vi "SLSC Get EDS Module Information_O2.vi"(5 "Password":string, 7 "Username":string="admin", 8 "error in (no error)":errorcluster, 10 "Slot #":u32=6, 11 "Chassis IP Address":string="192.168.8.130") -> (0 "error out":errorcluster, 1 "SLSC Module Name":string, 2 "Initialized?":bool, 3 "SLSC EDS module":T1)   [LabVIEW 2017]
doc: "This vi reads device tree from online SLSC module. If there is no connection possible it reads from a capabilities NVMEM .bin file. Then it creates a cluster containing the whole module tree."
uses:
  SLSC EDS API/JSON parsing/EDSjsonStructure.ctl
  SLSC EDS API/JSON parsing/enum.ctl
  SLSC EDS API/JSON parsing/property.ctl
  SLSC EDS API/JSON parsing/command.ctl
  SLSC EDS API/JSON parsing/scale.ctl
  SLSC EDS API/JSON parsing/physicalChannel.ctl
  SLSC EDS API/JSON parsing/register.ctl
  SLSC EDS API/SLSC EDS API.lvlib
panel:
  # "not working\nregisterMap->registers->initialValue"
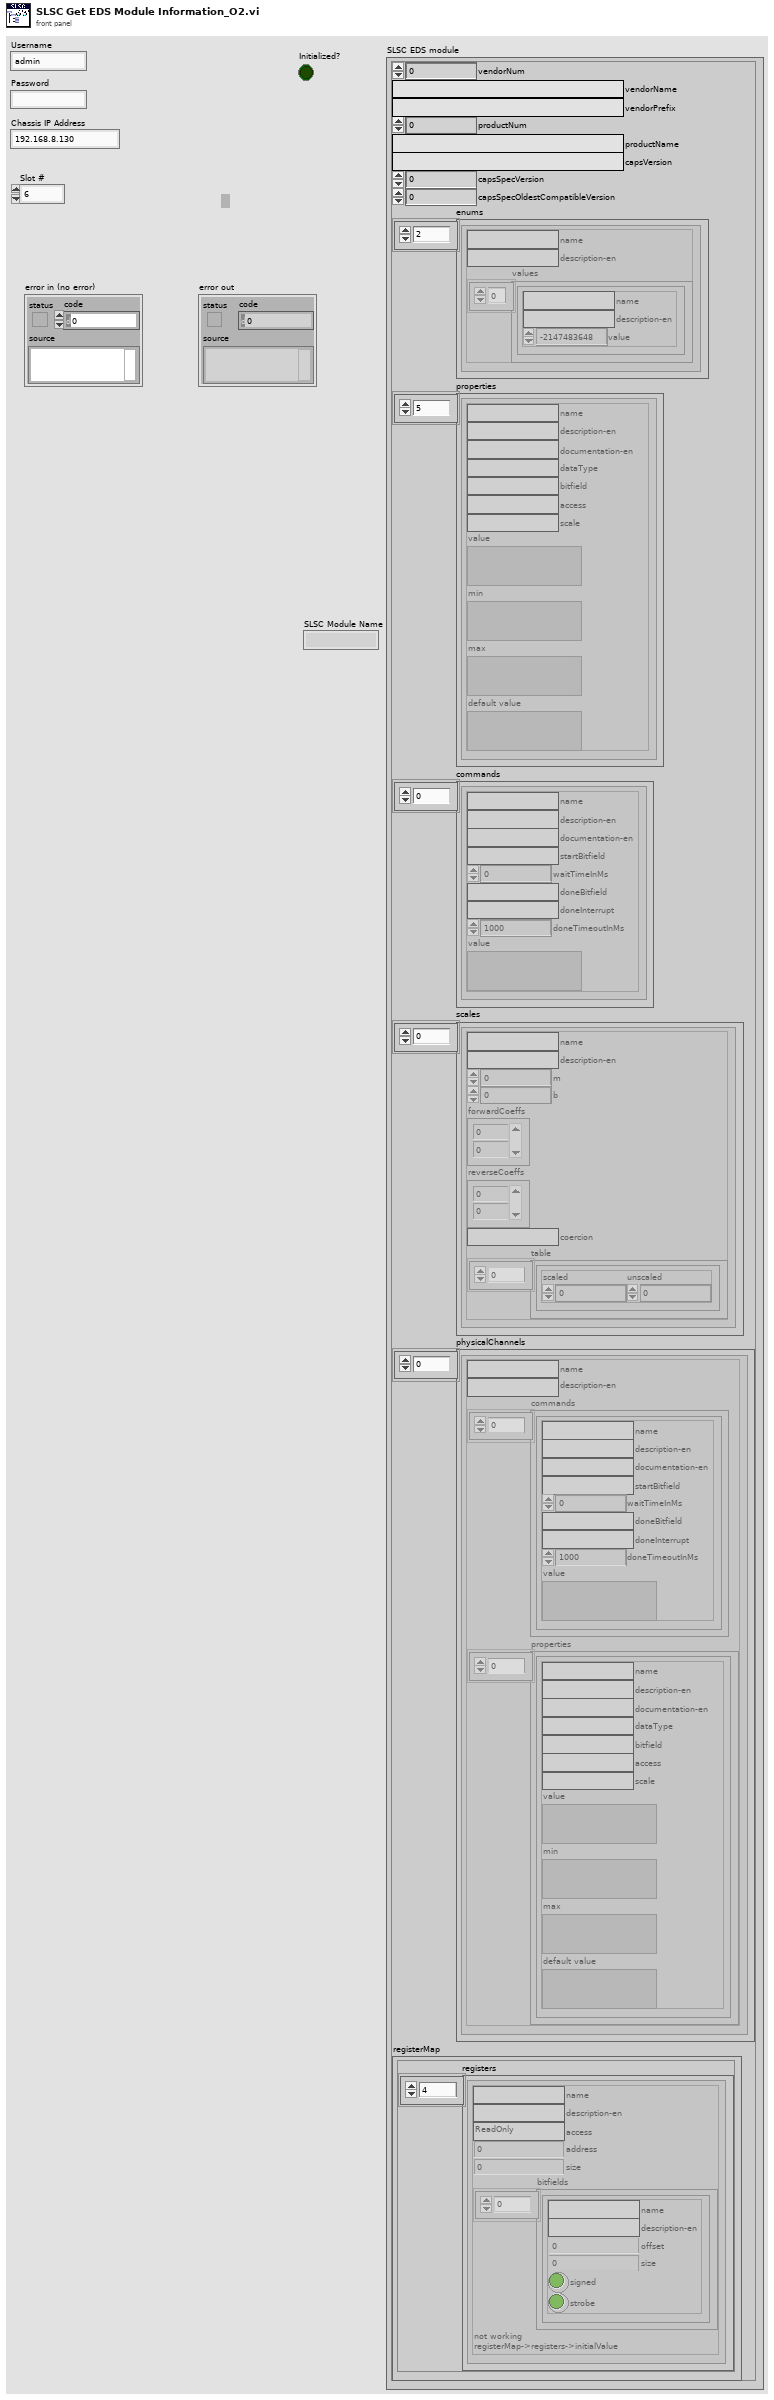
[diagram p1: front panel]
types:
  T1 = typedef "EDSjsonStructure.ctl" = cluster{"vendorNum":u32, "vendorName":string, "vendorPrefix":string, "productNum":u32, "productName":string, "capsVersion":string, "capsSpecVersion":u32, "capsSpecOldestCompatibleVersion":u32, "enums":T2[], "properties":T3[], "commands":T4[], "scales":T5[], "physicalChannels":T6[], "registerMap":cluster{"registers":T7[]}}
  T2 = typedef "enum.ctl" = cluster{"name":string, "description-en":string, "values":cluster{"name":string, "description-en":string, "value":i32}[]}
  T3 = typedef "property.ctl" = cluster{"name":string, "description-en":string, "documentation-en":string, "dataType":string, "bitfield":string, "access":string, "scale":string, "value":variant, "min":variant, "max":variant, "default value":variant}
  T4 = typedef "command.ctl" = cluster{"name":string, "description-en":string, "documentation-en":string, "startBitfield":string, "waitTimeInMs":i32, "doneBitfield":string, "doneInterrupt":string, "doneTimeoutInMs":i32, "value":variant}
  T5 = typedef "scale.ctl" = cluster{"name":string, "description-en":string, "m":dbl, "b":dbl, "forwardCoeffs":dbl[], "reverseCoeffs":dbl[], "coercion":string, "table":cluster{"scaled":dbl, "unscaled":dbl}[]}
  T6 = typedef "physicalChannel.ctl" = cluster{"name":string, "description-en":string, "commands":T4[], "properties":T3[]}
  T7 = typedef "register.ctl" = cluster{"name":string, "description-en":string, "access":string, "address":u32, "size":u32, "bitfields":cluster{"name":string, "description-en":string, "offset":u32, "size":u32, "signed":bool, "strobe":bool}[]}
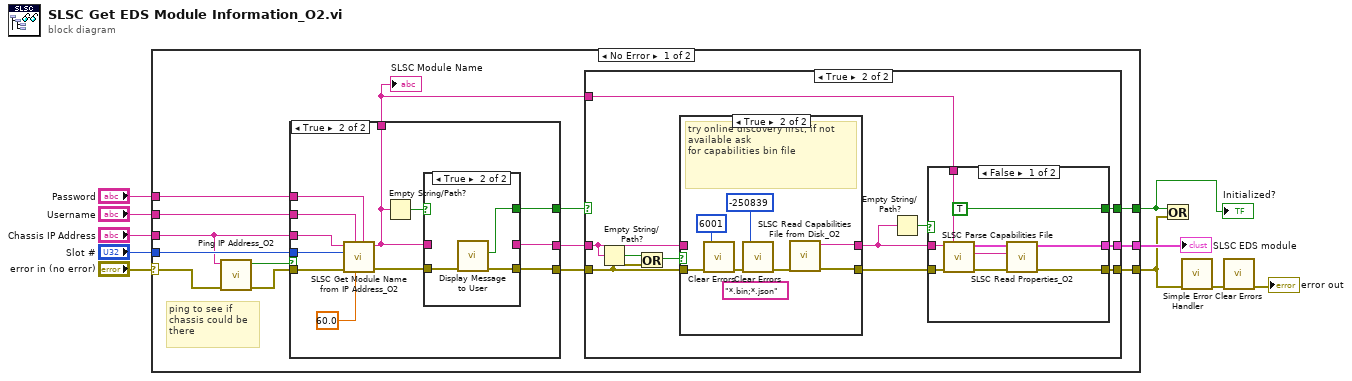
[diagram p0: block diagram]
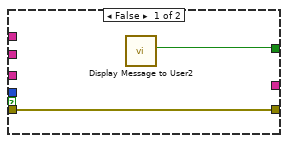
[diagram p5: hidden frame]
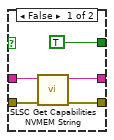
[diagram p6: hidden frame]
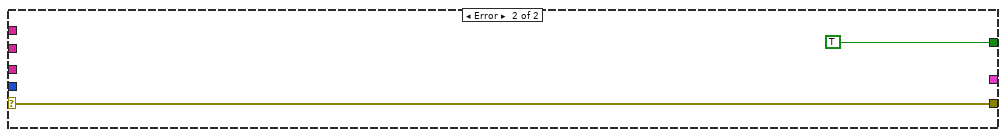
[diagram p7: hidden frame]
diagram:
  n1 = case shown="No Error" "error in (no error)" {
    selector: "error in (no error)" -> [w21 w78]
    tunnel: [w14 w78] -> w4
    tunnel: "Chassis IP Address" -> [w20 _]
    tunnel: "Slot #" -> [w24 _]
    tunnel: "Username" -> [w23 _]
    tunnel: "Password" -> [w22 _]
    tunnel: [w15 _] -> w5
    tunnel: [w11 TRUE ("Failed?")] -> w1
    frame No Error {
      # "ping to see if \nchassis could be \nthere"
      n2 = call "Ping IP Address_O2.vi"("error in"=w21, "host"=w20) -> ("error out"=w19:errorcluster, "response?"=w18:bool)  [unwired: 7 in, 1 out]
      n3 = case shown="True" w18 {
        tunnel: w19 -> [w55 w59]
        tunnel: w20 -> [_ w65]
        tunnel: w24 -> [_ w64]
        tunnel: w23 -> [_ w67]
        tunnel: w22 -> [_ w66]
        tunnel: [w55 w63] -> w17
        tunnel: [_ w61] -> w16
        tunnel: [_ w58] -> w13
        tunnel: [w56 w60] -> w12
        frame False {
          n4 = call "Display Message to User2"() -> ("Yes"=w56:bool)  [unwired: 10 in, 1 out]
        }
        frame True {
          n5 = call "SLSC Get Module Name from IP Address_O2.vi"("Password"=w66, "connect timeout"=60.0 ("connect timeout (10 sec)"), "Username"=w67, "Error In"=w59, "Slot #"=w64, "Chassis IP Address"=w65) -> ("Error Out"=w57:errorcluster, "SLSC Module Name"=w58:string)  [unwired: 3 in, 1 out]
          n6 = Empty String/Path?(string/path=w58) -> (empty?=w62:bool)
          n7 = case shown="True" w62 {
            tunnel: w57 -> [w73 w76]
            tunnel: [w72 w75] -> w63
            tunnel: [w71 _] -> w61
            tunnel: w58 -> [w70 _]
            tunnel: [TRUE ("Yes") w74] -> w60
            frame False {
              n8 = call "SLSC Get Capabilities NVMEM String.vi"("error in (no error)"=w73, "SLSC Device"=w70) -> ("error out"=w72:errorcluster, "capabilities NVMEM"=w71:string)  [unwired: 8 in]
            }
            frame True {
              n9 = call "Display Message to User"("error in (no error)"=w76) -> ("error out"=w75:errorcluster, "Yes"=w74:bool)  [unwired: 9 in]
            }
          }
        }
      }
      "SLSC Module Name" <- w13
      n10 = case shown="True" w12 {
        tunnel: w17 -> [w25 w31]
        tunnel: w16 -> [_ w30]
        tunnel: [_ w35] -> w15
        tunnel: [w25 w34] -> w14
        tunnel: w13 -> [_ w33]
        tunnel: [_ w26] -> w11
        frame False {
        }
        frame True {
          n11 = Empty String/Path?(string/path=w30) -> (empty?=w29:bool)
          n12 = Or(x=w29, y=w31) -> (x .or. y?=w32:bool)
          n13 = case shown="True" w32 {
            tunnel: [w46 w49] -> w36
            tunnel: w30 -> [w47 _]
            tunnel: [w47 w48] -> w28
            tunnel: w31 -> [w46 w51]
            frame False {
            }
            frame True {
              (unwired) "*.bin;*.json" ("pattern (all files)")
              # "try online discovery first, if not available ask \nfor capabilities bin file"
              n14 = call <vilib>:"Clear Errors.vi"("error in (no error)"=w51, "specific error code to clear (0: all)"=6001) -> ("error out"=w52:errorcluster)  [unwired: 4 in, 1 out]
              n15 = call <vilib>:"Clear Errors.vi"("error in (no error)"=w52, "specific error code to clear (0: all)"=-250839) -> ("error out"=w50:errorcluster)  [unwired: 4 in, 1 out]
              n16 = call "SLSC Read Capabilities File from Disk_O2.vi"("error in (no error)"=w50) -> ("error out"=w49:errorcluster, "String"=w48:string)  [unwired: 9 in]
            }
          }
          n17 = Empty String/Path?(string/path=w28) -> (empty?=w27:bool)
          n18 = case shown="False" w27 {
            tunnel: w36 -> [w44 w45]
            tunnel: [w41 _] -> w35
            tunnel: [w40 w45] -> w34
            tunnel: w33 -> [w37 _]
            tunnel: w28 -> [w39 _]
            tunnel: [TRUE _] -> w26
            frame False {
              n19 = call "SLSC Parse Capabilities File.vi"("error in"=w44, "module capabilities JSON string"=w39) -> ("error out"=w42:errorcluster, "SLSC EDS module"=w43:T1)  [unwired: 8 in]
              n20 = call "SLSC Read Properties_O2.vi"("error in (no error)"=w42, "SLSC Device"=w37, "SLSC EDS module in"=w43) -> ("error out"=w40:errorcluster, "SLSC EDS module out"=w41:T1)  [unwired: 7 in]
            }
            frame True {
            }
          }
        }
      }
    }
    frame Error {
    }
  }
  "SLSC EDS module" <- w5
  "Initialized?" <- w1
  n21 = Or(x=w1, y=w4) -> ()  [unwired: 1 out]
  n22 = call <vilib>:"Simple Error Handler.vi"("error in (no error)"=w4) -> ("error out"=w3:errorcluster)  [unwired: 4 in, 4 out]
  n23 = call <vilib>:"Clear Errors.vi"("error in (no error)"=w3) -> ("error out"=→"error out":errorcluster)  [unwired: 5 in, 1 out]
